vi "探头窗口-16-网络版.vi"() -> ()   [LabVIEW 2017]
panel:
  in  "外部停止命令？":bool=TRUE
  out "引用-监测模式？":refnum<vi>
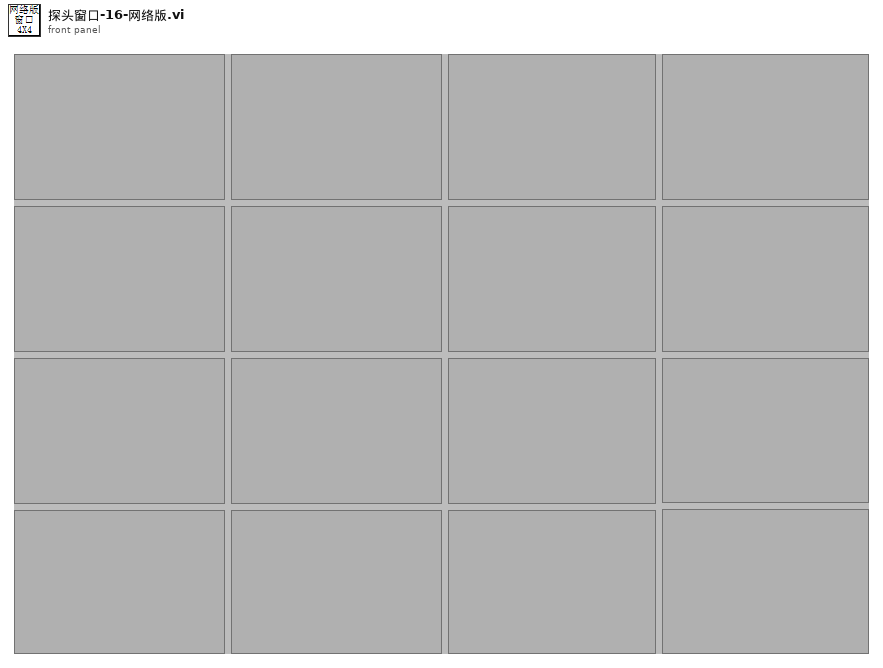
[diagram p1: front panel]
types:
  T1 = typedef "eventvkey.ctl" = enum16{"ASCII", "Enter", "Return", "Shift", "Ctrl", "Alt", "Cmd", "Opt", "Caps", "NumLock", "Clear", "Break", "Up", "Down", "Left", "Right", "Insert", "Delete", "Home", "End", "PageUp", "PageDown", "Escape", "Help", "Pause", "ScrollLock", "F1", "F2", "F3", "F4", "F5", "F6", "F7", "F8", "F9", "F10", "F11", "F12", "F13", "F14", "F15", "F16", "F17", "F18", "F19", "F20", "F21", "F22", "F23", "F24", "Play", "VolumeUp", "VolumeDown", "Mute", "Two Byte Char"}
  T2 = typedef "探头属性.ctl" = cluster{"探头地址与信息":T3, "测量值":T6, "限值":T7, "探头状态":T8, "累积记录":T9, "报警方式":T10}
  T3 = typedef "探测器信息.ctl" = cluster{"网络地址":string, "名称":string, "备注":string, "累积剂量":dbl, "累积限值":dbl, "硬件剂量率限值":T4, "剂量率限值1":dbl, "剂量率限值2":dbl, "报警方式":T5}
  T4 = typedef "探头剂量率限值选择.ctl" = enum16{"一级限值", "二级限值"}
  T5 = typedef "报警方式选择.ctl" = enum16{"常报警", "自动静音", "手动静音"}
  T6 = typedef "测量值.ctl" = cluster{"时间":timestamp, "数值":dbl}
  T7 = typedef "剂量率限值.ctl" = cluster{"限值1":dbl, "限值2":dbl, "探头限值":T4}
  T8 = typedef "探头状态.ctl" = enum16{"正常", "离线", "禁用", "一级报警", "二级报警", "累积报警"}
  T9 = typedef "单条累积记录.ctl" = cluster{"起始时间":timestamp, "结束时间":timestamp, "累积剂量":dbl}
  T10 = typedef "报警方式.ctl" = cluster{"报警方式":T5, "延迟计时":u16, "报警中？":bool}
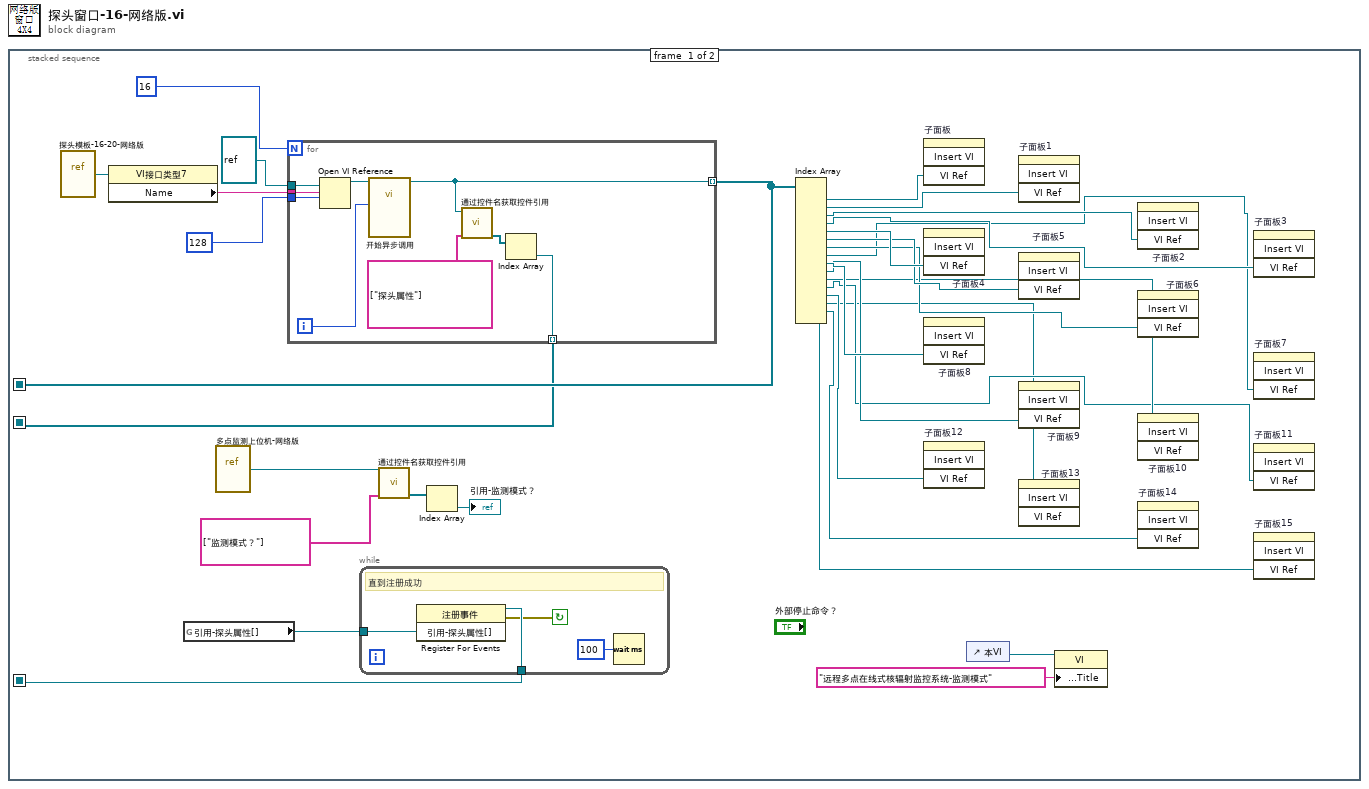
[diagram p0: block diagram]
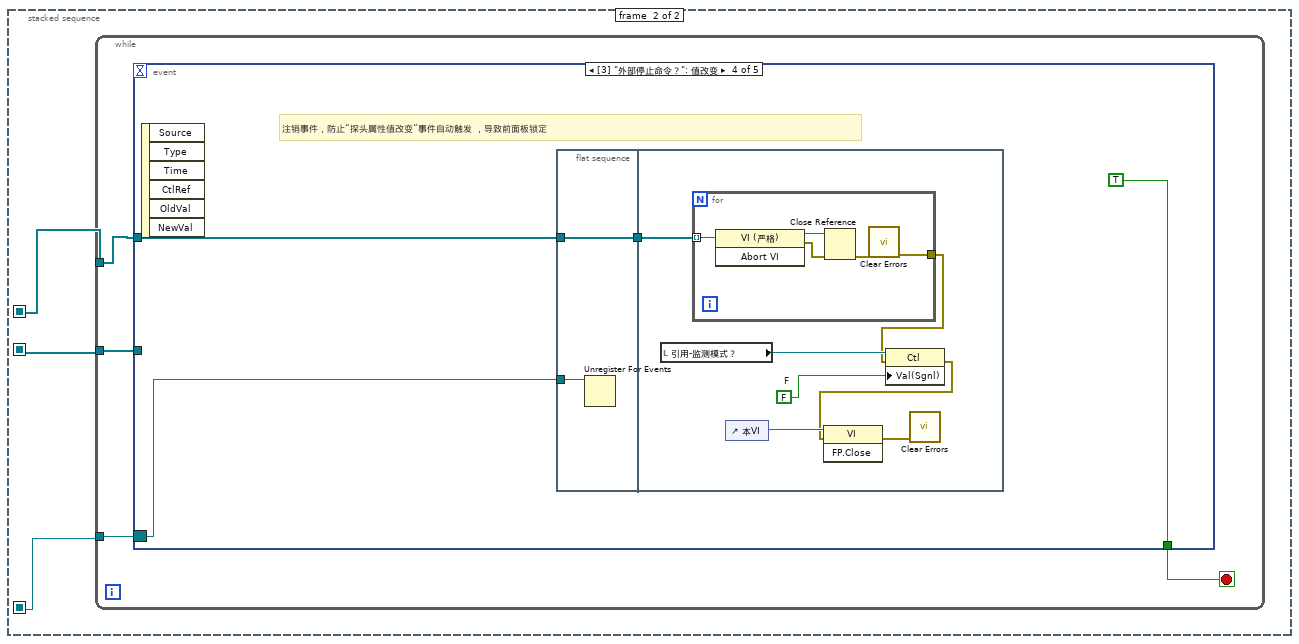
[diagram p2: hidden frame]
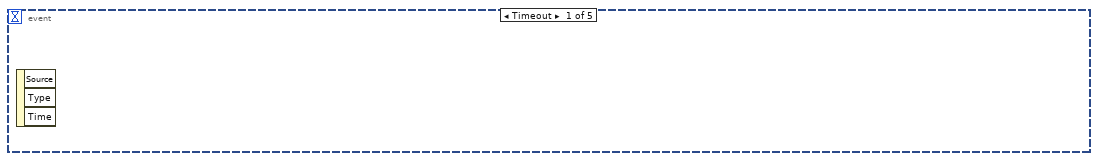
[diagram p3: hidden frame]
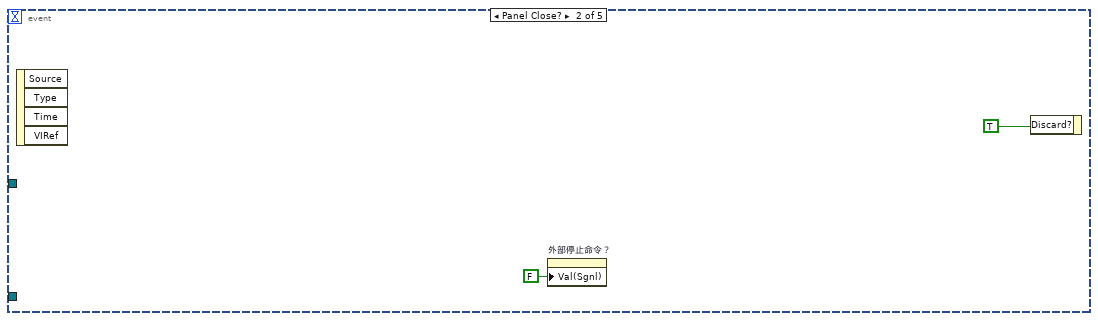
[diagram p4: hidden frame]
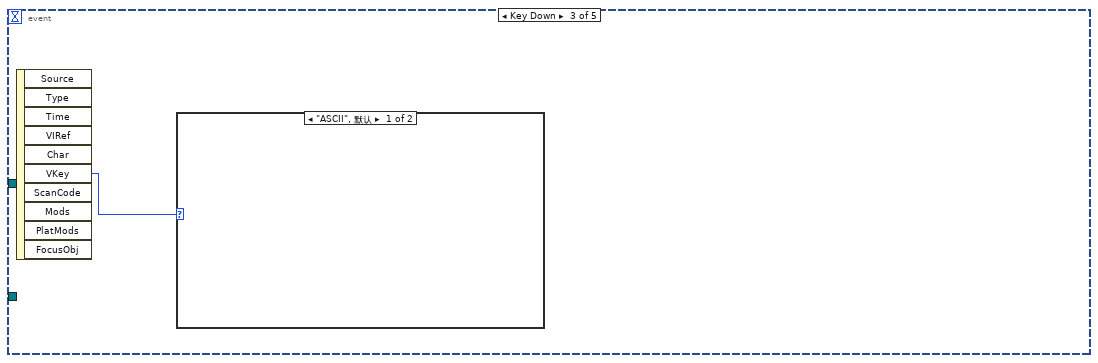
[diagram p5: hidden frame]
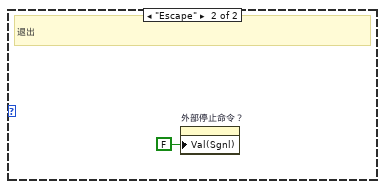
[diagram p6: hidden frame]
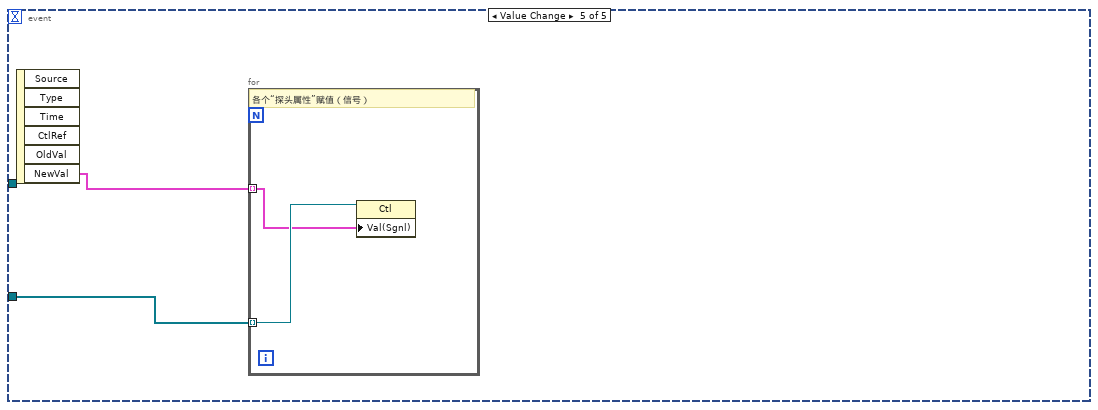
[diagram p7: hidden frame]
diagram:
  n1 = stacked-sequence {
    seq-local: [w30 _] -> [_ w47]
    seq-local: [w9 _] -> [_ w46]
    seq-local: [w1 _] -> [_ w45]
    frame #0 {
      n2 = vi-ref "探头模板-16-20-网络版.vi"() -> (w6:refnum<vi>)
      n3 = property class="VI接口类型7"(reference=w6) -> ("Name"=w5:string)  [unwired: 1 in, 2 out]
      n4 = global read "全局变量-35点监测.vi" "引用-探头属性[]"() -> (w2:refnum<vi>)
      n5 = vi-ref "多点监测上位机-网络版.vi"() -> (w10:refnum<vi>)
      n6 = for "For循环" {
        N: 16 -> [_]
        tunnel: w5 -> [w44]
        tunnel: 128 ("选项") -> [w43]
        tunnel: refnum<vi> refnum ("类型说明符VI引用句柄（仅用于类型）") -> [w42]
        tunnel: [w37] -> w30 mode=indexing
        tunnel: [w38] -> w9 mode=indexing
        i -> [w36]
        n7 = Open VI Reference(type specifier VI Refnum (for type only)=w42, vi path=w44, options=w43) -> (vi reference=w39:refnum<vi>)  [unwired: 3 in, 1 out]
        n8 = call-by-ref "开始异步调用"(reference=w39, "探头序号"=w36) -> (reference out=w37:refnum<vi>)  [unwired: 12 in, 1 out]
        n9 = call "通过控件名获取控件引用.vi"("控件名数组"=string[] ["探头属性"], "VI引用"=w37) -> ("控件引用输出"=w41:refnum<vi>[])  [unwired: 7 in, 2 out]
        n10 = Index Array(array=w41) -> (element=w38:refnum<vi>)  [unwired: 1 in]
      }
      n11 = while {
        tunnel: w2 -> [w35]
        tunnel: [w34] -> w1
        stop <- w33 continue-if-true
        # "直到注册成功"
        n12 = register-events(w35) -> (reference out=w34:refnum<event-registration>, error out=w33:errorcluster)  [unwired: 2 in]
        n13 = Wait (ms)(milliseconds to wait=u32 100 ("等待时间（毫秒）")) -> ()  [unwired: 1 out]
      }
      n14 = call "通过控件名获取控件引用.vi"("控件名数组"=string[] ["监测模式？"], "VI引用"=w10) -> ("控件引用输出"=w12:refnum<vi>[])  [unwired: 7 in, 2 out]
      n15 = Index Array(array=w12) -> (element=→"引用-监测模式？":refnum<vi>)  [unwired: 1 in]
      n16 = Index Array(array=w30) -> (element #1=w29:refnum<vi>, element #2=w28:refnum<vi>, element #3=w27:refnum<vi>, element #4=w26:refnum<vi>, element #5=w25:refnum<vi>, element #6=w24:refnum<vi>, element #7=w23:refnum<vi>, element #8=w22:refnum<vi>, element #9=w21:refnum<vi>, element #10=w20:refnum<vi>, element #11=w19:refnum<vi>, element #12=w18:refnum<vi>, element #13=w17:refnum<vi>, element #14=w16:refnum<vi>, element #15=w15:refnum<vi>, element #16=w14:refnum<vi>)  [unwired: 16 in]
      n17 = invoke on="子面板" class="子面板" method="Insert VI"("VI Ref"=w29) -> ()  [unwired: 3 in, 4 out]
      n18 = invoke on="子面板4" class="SubPnl" method="Insert VI"("VI Ref"=w25) -> ()  [unwired: 3 in, 4 out]
      n19 = invoke on="子面板8" class="SubPnl" method="Insert VI"("VI Ref"=w21) -> ()  [unwired: 3 in, 4 out]
      n20 = invoke on="子面板12" class="SubPnl" method="Insert VI"("VI Ref"=w17) -> ()  [unwired: 3 in, 4 out]
      n21 = control-ref of="本VI"() -> (w8:refnum<vi>)
      n22 = invoke on="子面板1" class="SubPnl" method="Insert VI"("VI Ref"=w28) -> ()  [unwired: 3 in, 4 out]
      n23 = invoke on="子面板5" class="SubPnl" method="Insert VI"("VI Ref"=w24) -> ()  [unwired: 3 in, 4 out]
      n24 = invoke on="子面板9" class="SubPnl" method="Insert VI"("VI Ref"=w20) -> ()  [unwired: 3 in, 4 out]
      n25 = invoke on="子面板13" class="SubPnl" method="Insert VI"("VI Ref"=w16) -> ()  [unwired: 3 in, 4 out]
      n26 = property class="VI"(reference=w8, "Front Panel.Title"="远程多点在线式核辐射监控系统-监测模式" ("前面板窗口:标题")) -> ()  [unwired: 1 in, 2 out]
      n27 = invoke on="子面板2" class="SubPnl" method="Insert VI"("VI Ref"=w27) -> ()  [unwired: 3 in, 4 out]
      n28 = invoke on="子面板6" class="SubPnl" method="Insert VI"("VI Ref"=w23) -> ()  [unwired: 3 in, 4 out]
      n29 = invoke on="子面板10" class="SubPnl" method="Insert VI"("VI Ref"=w19) -> ()  [unwired: 3 in, 4 out]
      n30 = invoke on="子面板14" class="SubPnl" method="Insert VI"("VI Ref"=w15) -> ()  [unwired: 3 in, 4 out]
      n31 = invoke on="子面板3" class="SubPnl" method="Insert VI"("VI Ref"=w26) -> ()  [unwired: 3 in, 4 out]
      n32 = invoke on="子面板7" class="SubPnl" method="Insert VI"("VI Ref"=w22) -> ()  [unwired: 3 in, 4 out]
      n33 = invoke on="子面板11" class="SubPnl" method="Insert VI"("VI Ref"=w18) -> ()  [unwired: 3 in, 4 out]
      n34 = invoke on="子面板15" class="SubPnl" method="Insert VI"("VI Ref"=w14) -> ()  [unwired: 3 in, 4 out]
    }
    frame #1 {
      n35 = while {
        tunnel: w47 -> [w50]
        tunnel: w46 -> [w49]
        tunnel: w45 -> [w48]
        stop <- w51 stop-if-true
        n36 = event shown="[3] \"外部停止命令？\": 值改变" {
          selector: w48 -> [_ _ _ w56 _]
          dyn-events: _ -> [_ _ _ _ _]
          timeout: _ -> [_ _ _ _ _]
          tunnel: [_ _ _ TRUE ("放弃？") _] -> w51
          tunnel: w50 -> [_ _ _ w58 _]
          tunnel: w49 -> [_ _ _ _ w74]
          event Timeout {
            n37 = event-data() -> ()  [unwired: 1 in, 3 out]
          }
          event Panel Close? {
            n38 = event-data() -> ()  [unwired: 1 in, 4 out]
            n39 = property on="外部停止命令？" class="Bool (严格)"("Val(Sgnl)"=FALSE ("值(信号)")) -> ()  [unwired: 2 in, 2 out]
            n40 = event-data("Discard?"=TRUE ("放弃？")) -> ()  [unwired: 1 in, 1 out]
          }
          event Key Down {
            n41 = event-data() -> ("VKey"=w54:T1)  [unwired: 1 in, 9 out]
            n42 = case shown="\"ASCII\", 默认" w54 {
              frame "ASCII", Default {
              }
              frame "Escape" {
                # "退出"
                n43 = property on="外部停止命令？" class="Bool (严格)"("Val(Sgnl)"=FALSE ("值(信号)")) -> ()  [unwired: 2 in, 2 out]
              }
            }
          }
          event "外部停止命令？": Value Change {
            # "注销事件，防止“探头属性值改变”事件自动触发 ，导致前面板锁定"
            n44 = event-data() -> ()  [unwired: 1 in, 6 out]
            n45 = flat-sequence {
              tunnel: w58 -> [w61]
              tunnel: [w61] -> w57
              tunnel: w56 -> [w60]
              tunnel: w57 -> [w68]
              frame #0 {
                n46 = Unregister For Events(event registration refnum=w60) -> ()  [unwired: 1 in, 1 out]
              }
              frame #1 {
                w67 = FALSE  # F
                n47 = local read "引用-监测模式？"() -> (w66:refnum<vi>)
                n48 = for "For循环" {
                  tunnel: w68 -> [w73] mode=indexing
                  tunnel: [w69] -> w64
                  n49 = invoke class="VI (严格)" method="Abort VI"(reference=w73) -> (reference out=w71:refnum<vi>, error out=w72:errorcluster)  [unwired: 2 in, 1 out]
                  n50 = Close Reference(reference=w71, error in (no error)=w72) -> (error out=w70:errorcluster)
                  n51 = call <vilib>:"Clear Errors.vi"("error in (no error)"=w70) -> ("error out"=w69:errorcluster)  [unwired: 5 in, 1 out]
                }
                n52 = control-ref of="本VI"() -> (w65:refnum<vi>)
                n53 = property class="Ctl"(reference=w66, error in=w64, "Val(Sgnl)"=w67) -> (error out=w63:errorcluster)  [unwired: 1 out]
                n54 = invoke class="VI" method="FP.Close"(reference=w65, error in=w63) -> (error out=w62:errorcluster)  [unwired: 1 in, 2 out]
                n55 = call <vilib>:"Clear Errors.vi"("error in (no error)"=w62) -> ()  [unwired: 5 in, 2 out]
              }
            }
          }
          event Value Change {
            n56 = event-data() -> ("NewVal"=w75:T2[])  [unwired: 1 in, 5 out]
            n57 = for "For循环" {
              tunnel: w74 -> [w77] mode=indexing
              tunnel: w75 -> [w76] mode=indexing
              # "各个“探头属性”赋值（信号）"
              n58 = property class="Ctl"(reference=w77, "Val(Sgnl)"=w76) -> ()  [unwired: 1 in, 2 out]
            }
          }
        }
      }
    }
  }
